vi "Get Available Instances.vi"(4 "Error In":errorcluster) -> (0 "Error Out":errorcluster, 3 "Available Instances":string[](array[string]))   [LabVIEW 2020, in "Managing Executables.lvlib"]
uses:
  Managing Executables.lvlib
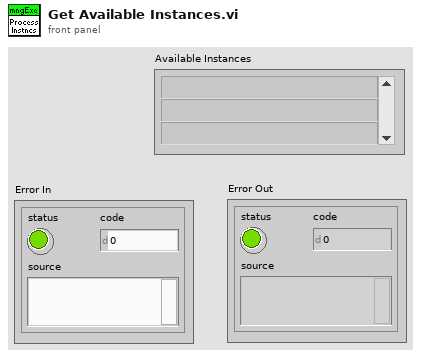
[diagram p1: front panel]
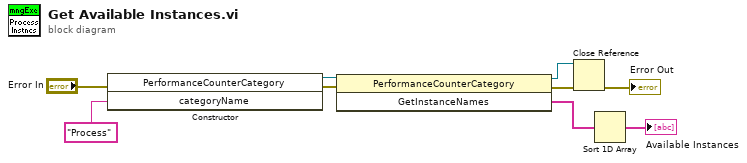
[diagram p0: block diagram]
diagram:
  n1 = constructor class="PerformanceCounterCategory"(error in="Error In", "categoryName"="Process" ("Category List 2")) -> (reference out=w8:refnum<k24>, error out=w7:errorcluster)  [unwired: 2 in, 2 out]
  n2 = invoke class="PerformanceCounterCategory" method="GetInstanceNames"(reference=w8, error in=w7) -> (reference out=w5:refnum<k24>, error out=w3:errorcluster, "GetInstanceNames"=w6:string[])  [unwired: 1 in]
  n3 = Close Reference(reference=w5, error in (no error)=w3) -> (error out=→"Error Out":errorcluster)
  n4 = Sort 1D Array(array=w6) -> (sorted array=→"Available Instances":string[])
